vi "SynchronizeClusters.vi"(6 "toSettings":bool, 7 "variant (destination)":variant, 8 "error in (no error)":errorcluster, 9 "Seperator (\"\")":string="Channel 1", 11 "variant  (source)":variant) -> (0 "error  out":errorcluster, 1 "Seperator out":string="Channel 1", 3 "variant out":variant)   [LabVIEW 2011]
panel:
  out "Array 2":string[](array[string])
  out "Array":string[](array[string])
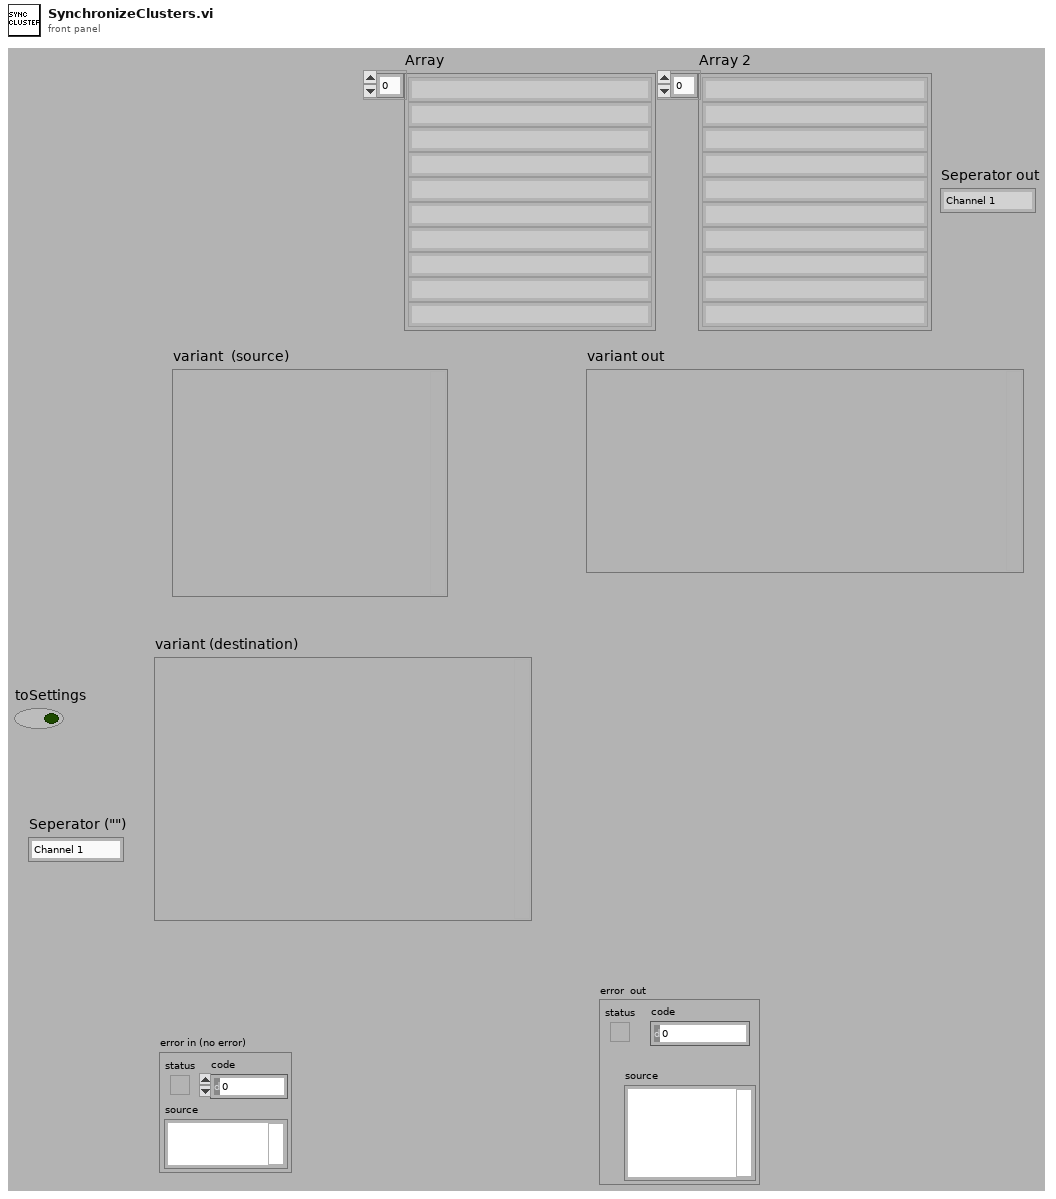
[diagram p1: front panel]
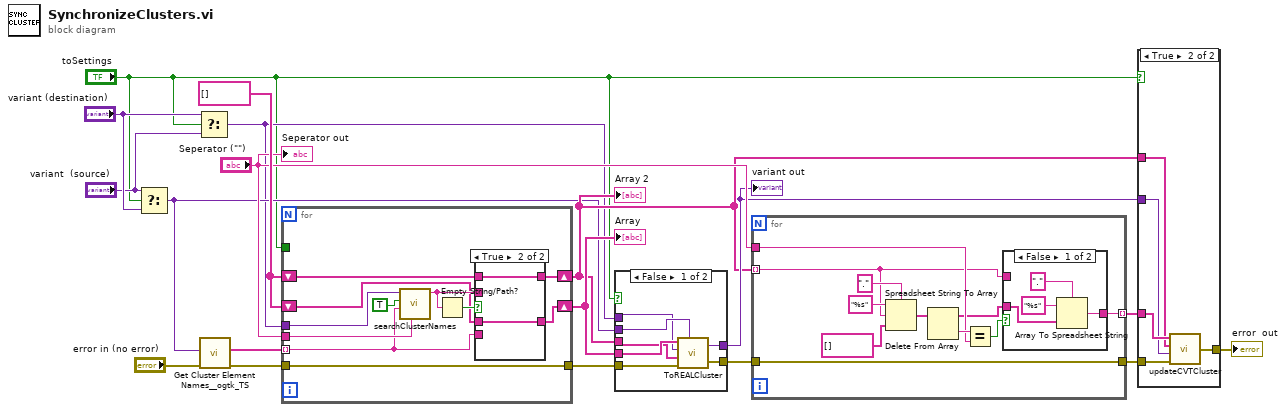
[diagram p0: block diagram]
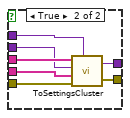
[diagram p4: hidden frame]
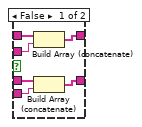
[diagram p5: hidden frame]
diagram:
  w17 = string[] []
  n1 = Select(t="variant  (source)", s="toSettings", f="variant (destination)") -> (s? t:f=w11:variant)
  n2 = Select(t="variant (destination)", s="toSettings", f="variant  (source)") -> (s? t:f=w10:variant)
  n3 = call "Get Cluster Element Names__ogtk_TS.vi"("error in (no error)"="error in (no error)", "Variant"=w11) -> ("error out"=w5:errorcluster, "Names (Array)"=w18:string[])  [unwired: 8 in]
  n4 = for {
    tunnel: w18 -> [w23] mode=indexing
    tunnel: w10 -> [w29]
    tunnel: "Seperator (\"\")" -> [w28]
    shift-right: [w26] -> w12
    shift-left: w17 -> [w25]
    shift-right: [w21] -> w16
    shift-left: w17 -> [w22]
    tunnel: "toSettings" -> [_]
    tunnel: w5 -> [w19]
    tunnel: [w19] -> w4
    n5 = call "searchClusterNames.vi"("Separator (\"\") 2"=w28, "Command or variable"=w23, "exact match"=TRUE, "variant (destination) 2"=w29) -> ("element"=w27:string)  [unwired: 6 in, 1 out]
    n6 = Empty String/Path?(string/path=w27) -> (empty?=w24:bool)
    n7 = case shown="True" w24 {
      tunnel: w27 -> [w35 _]
      tunnel: [w34 w37] -> w26
      tunnel: w25 -> [w33 w37]
      tunnel: w23 -> [w32 _]
      tunnel: w22 -> [w31 w36]
      tunnel: [w30 w36] -> w21
      frame False {
        n8 = Build Array (concatenate)(w33, w35) -> (w34:string[])
        n9 = Build Array (concatenate)(w31, w32) -> (w30:string[])
      }
      frame True {
      }
    }
  }
  "Array" <- w16
  "Array 2" <- w12
  n10 = case shown="False" "toSettings" {
    tunnel: w12 -> [w41 w51]
    tunnel: w11 -> [w40 w50]
    tunnel: w10 -> [w39 w49]
    tunnel: w16 -> [w42 w48]
    tunnel: [w44 w47] -> w13
    tunnel: w4 -> [w38 w45]
    tunnel: [w43 w46] -> w3
    frame False {
      n11 = call "ToREALCluster.vi"("Element Names (destination) out"=w42, "variant  (source)"=w39, "Array"=w41, "error out"=w38, "variant (destination)"=w40) -> ("variant (destination) out"=w44:variant, "error out 2"=w43:errorcluster)
    }
    frame True {
      n12 = call "ToSettingsCluster.vi"("Element Names (destination) out"=w51, "variant  (source)"=w50, "Element Names (source)"=w48, "error out"=w45, "variant (destination)"=w49) -> ("variant (destination) out"=w47:variant, "error out 2"=w46:errorcluster)
    }
  }
  "variant out" <- w13
  n13 = for {
    tunnel: w12 -> [w55] mode=indexing
    tunnel: "Seperator (\"\")" -> [w57]
    tunnel: [w54] -> w14 mode=indexing
    tunnel: w3 -> [w52]
    tunnel: [w52] -> w2
    n14 = Spreadsheet String To Array(delimiter (Tab)=".", format string="%s", spreadsheet string=w55, array type (2D Dbl)=string[] []) -> (array=w59:string[])
    n15 = Delete From Array(array=w59) -> (deleted portion=w58:string, array with subset deleted=w53:string[])  [unwired: 2 in]
    n16 = Equal?(x=w58, y=w57) -> (x = y?=w56:bool)
    n17 = case shown="False" w56 {
      tunnel: w55 -> [_ w67]
      tunnel: [w63 w67] -> w54
      tunnel: w53 -> [w66 _]
      frame False {
        n18 = Array To Spreadsheet String(delimiter (Tab)=".", array=w66, 3:"%s" ("format string")) -> (spreadsheet string=w63:string)
      }
      frame True {
      }
    }
  }
  n19 = case shown="True" "toSettings" {
    tunnel: w14 -> [_ w73]
    tunnel: w12 -> [_ w72]
    tunnel: w13 -> [_ w71]
    tunnel: w2 -> [w68 w70]
    tunnel: [w68 w69] -> w1
    frame False {
    }
    frame True {
      n20 = call "updateCVTCluster.vi"("error in"=w70, "variant (destination) out"=w71, "Cluster Names"=w72, "CVT Names"=w73) -> ("error out"=w69:errorcluster)
    }
  }
  "error  out" <- w1
  "Seperator out" <- "Seperator (\"\")"
